vi "parseFullEngineeringStatus.vi"(8 "error in (no error)":errorcluster, 10 "engineeringStatusString":string, 11 "DomeCommunicator in":refnum<class "ATDomeCommunicator.lvclass">) -> (0 "error out":errorcluster, 2 "fullEngineeringStatus":T1 {"shortStatus"."azimuthAngle" min=0.0 max=360.0; "shortStatus"."dropoutDoorOpeningPercentage" min=0.0 max=100.0; "shortStatus"."mainDoorOpeningPercentage" min=0.0 max=100.0}, 3 "DomeCommunicator out":refnum<class "ATDomeCommunicator.lvclass">)   [LabVIEW 2016, in "ATDomeCommunicator.lvclass"]
uses:
  ATDomeCommunicator.lvclass
  ComTypedefs/fullEngineeringStatus.ctl
  ComTypedefs/shortStatus.ctl
  ComTypedefs/openingStates.ctl
  IDome/domeTypedefs/openingPercentage.ctl
  ComTypedefs/sensorCode.ctl
  ComTypedefs/azimimuthPositionStatus.ctl
  IDome/domeTypedefs/azimuth.ctl
  IDome/domeTypedefs/direction.ctl
  IDome/domeTypedefs/domeState.ctl
  IDome/domeTypedefs/motionDirection.ctl
  IDome/domeTypedefs/openingMotion.ctl
  ComTypedefs/engineeringStatus.ctl
  <vilib>/regexp/Match Regular Expression.xnode
panel:
  out "after match":string
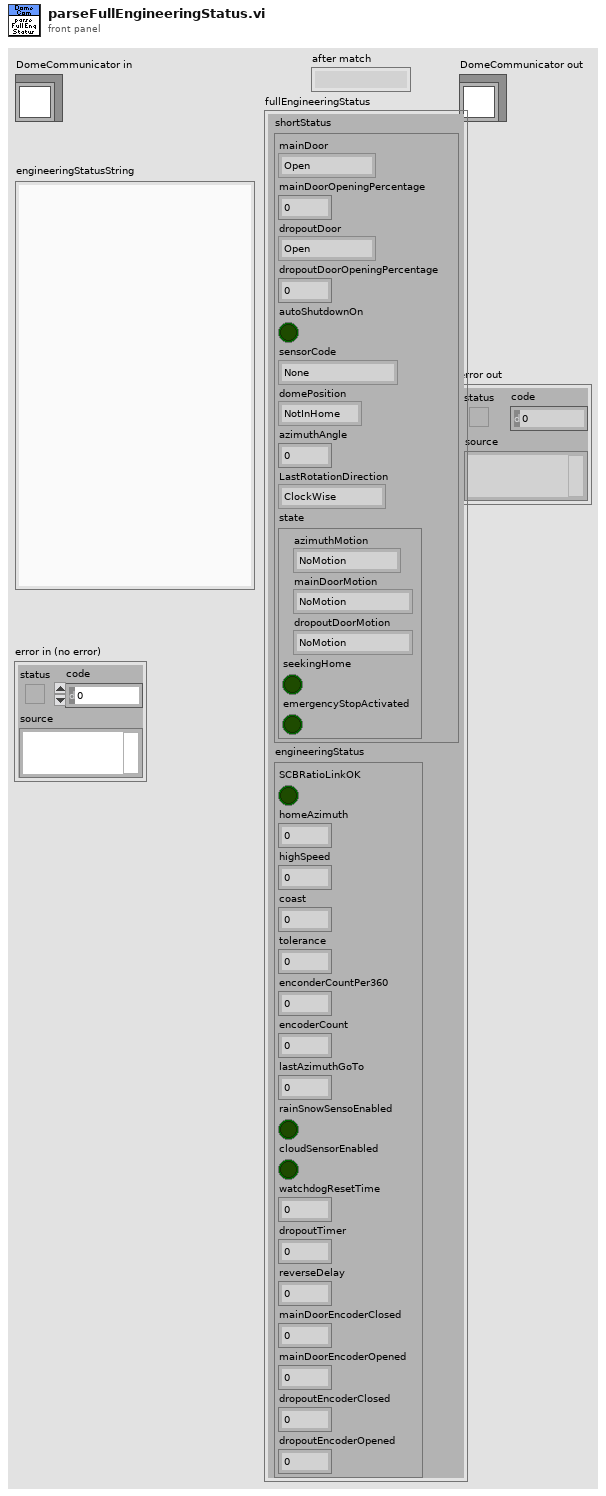
[diagram p1: front panel]
types:
  T1 = typedef "fullEngineeringStatus.ctl" = cluster{"shortStatus":T2, "engineeringStatus":T12}
  T2 = typedef "shortStatus.ctl" = cluster{"mainDoor":T3, "mainDoorOpeningPercentage":T4, "dropoutDoor":T3, "dropoutDoorOpeningPercentage":T4, "autoShutdownOn":bool, "sensorCode":T5, "domePosition":T6, "azimuthAngle":T7, "LastRotationDirection":T8, "state":T9}
  T3 = typedef "openingStates.ctl" = enum16{"Open", "Shut", "Ajar"}
  T4 = typedef "openingPercentage.ctl" = dbl
  T5 = typedef "sensorCode.ctl" = enum16{"None", "RainSnowSensorTriggered", "CloudSensorTriggered", "BothSensorsTriggered"}
  T6 = typedef "azimimuthPositionStatus.ctl" = enum16{"NotInHome", "Home"}
  T7 = typedef "azimuth.ctl" = dbl
  T8 = typedef "direction.ctl" = enum16{"ClockWise", "CounterClockWise"}
  T9 = typedef "domeState.ctl" = cluster{"azimuthMotion":T10, "mainDoorMotion":T11, "dropoutDoorMotion ":T11, "seekingHome":bool, "emergencyStopActivated":bool}
  T10 = typedef "motionDirection.ctl" = enum16{"NoMotion", "MovingClockWise", "MovingCounterClockWise"}
  T11 = typedef "openingMotion.ctl" = enum16{"NoMotion", "Opening", "Closing"}
  T12 = typedef "engineeringStatus.ctl" = cluster{"SCBRatioLinkOK":bool, "homeAzimuth":dbl, "highSpeed":dbl, "coast":dbl, "tolerance":dbl, "enconderCountPer360":u32, "encoderCount":u32, "lastAzimuthGoTo":dbl, "rainSnowSensoEnabled":bool, "cloudSensorEnabled":bool, "watchdogResetTime":dbl, "dropoutTimer":dbl, "reverseDelay":dbl, "mainDoorEncoderClosed":u32, "mainDoorEncoderOpened":u32, "dropoutEncoderClosed":u32, "dropoutEncoderOpened":u32}
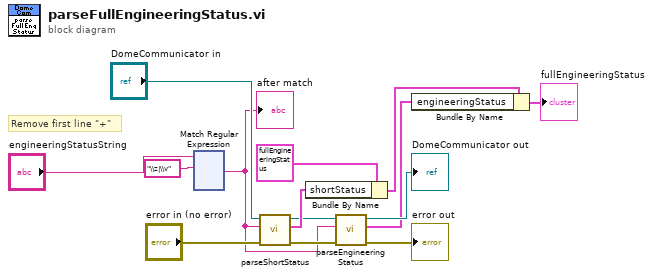
[diagram p0: block diagram]
diagram:
  # "Remove first line \"+\""
  n1 = xnode "Match Regular Expression"("input string"="engineeringStatusString", "regular expression"="\\z|\\v") -> ("after match"=w1:string)  [unwired: 4 in, 4 out]
  "after match" <- w1
  n2 = call "parseShortStatus.vi"("error in (no error)"="error in (no error)", "shortStatusString"=w1, "DomeCommunicator in"="DomeCommunicator in") -> ("error out"=w3:errorcluster, "shortStatus out"=w9:T2, "DomeCommunicator out"=w7:refnum<class "ATDomeCommunicator.lvclass">)  [unwired: 6 in]
  n3 = Bundle By Name(cluster=T1 {"shortStatus"={"mainDoor"=enum."Open", "mainDoorOpeningPercentage"=0.0, "dropoutDoor"=enum."Open", "dropoutDoorOpeningPercentage"=0.0, "autoShutdownOn"=FALSE, "sensorCode"=enum."None", "domePosition"=enum."NotInHome", "azimuthAngle"=0.0, "LastRotationDirection"=enum."ClockWise", "state"={"azimuthMotion"=enum."NoMotion", "mainDoorMotion"=enum."NoMotion", "dropoutDoorMotion "=enum."NoMotion", "seekingHome"=FALSE, "emergencyStopActivated"=FALSE}}, "engineeringStatus"={"SCBRatioLinkOK"=FALSE, "homeAzimuth"=0.0, "highSpeed"=0.0, "coast"=0.0, "tolerance"=0.0, "enconderCountPer360"=0, "encoderCount"=0, "lastAzimuthGoTo"=0.0, "rainSnowSensoEnabled"=FALSE, "cloudSensorEnabled"=FALSE, "watchdogResetTime"=0.0, "dropoutTimer"=0.0, "reverseDelay"=0.0, "mainDoorEncoderClosed"=0, "mainDoorEncoderOpened"=0, "dropoutEncoderClosed"=0, "dropoutEncoderOpened"=0}} ("FullEngineeringStatus"), "shortStatus"=w9) -> (w8:T1)
  n4 = call "parseEngineeringStatus.vi"("error in (no error)"=w3, "engineeringStatusString"=w1, "DomeCommunicator in"=w7) -> ("error out"=→"error out":errorcluster, "engineeringStatus"=w5:T12, "DomeCommunicator out"=→"DomeCommunicator out":refnum<class "ATDomeCommunicator.lvclass">)  [unwired: 6 in]
  n5 = Bundle By Name(cluster=w8, "engineeringStatus"=w5) -> (→"fullEngineeringStatus":T1)
